vi "InitPIC.vi"(4 "error in (no error)":errorcluster, 6 "DeviceKey In":string, 7 "CmdLib In":refnum<k24>) -> (0 "error out":errorcluster, 1 "Device Address Out":i32, 2 "DeviceKey Out":string, 3 "CmdLib Out":refnum<k24>)   [LabVIEW 2018]
uses:
  Device VIs/CmdLib.dll
  Device VIs/Verbal.vi
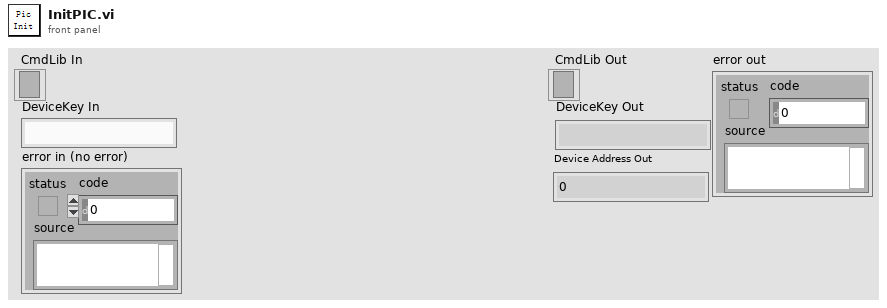
[diagram p1: front panel]
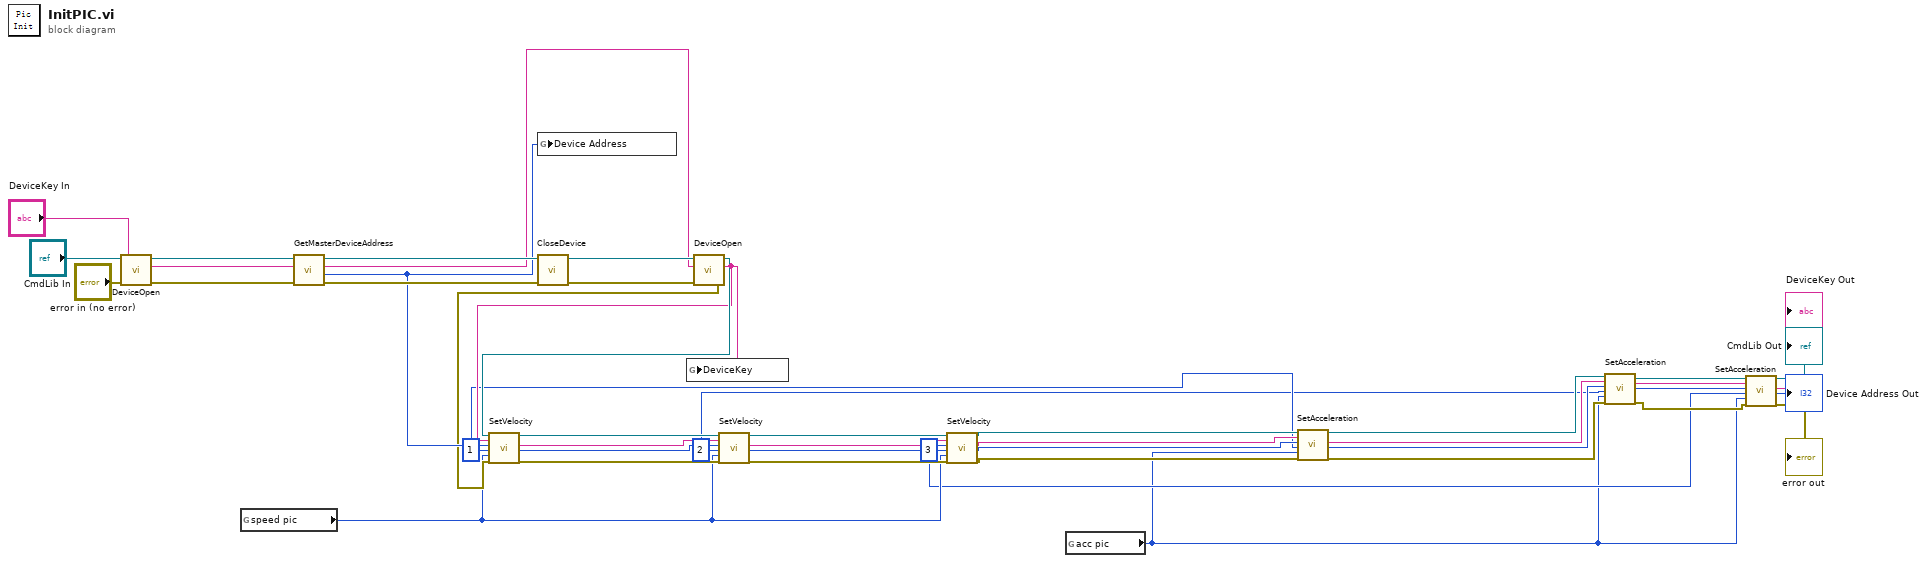
[diagram p0: block diagram]
diagram:
  w9 = 3 ("Motor")
  w14 = 2 ("Motor")
  w15 = 1 ("Motor")
  n1 = call "DeviceOpen.vi"("error in (no error)"="error in (no error)", "DeviceKey In"="DeviceKey In", "CmdLib In"="CmdLib In") -> ("error out"=w41:errorcluster, "DeviceKey Out"=w38:string, "CmdLib Out"=w42:refnum<k24>)  [unwired: 2 in]
  n2 = global read "Verbal.vi" "speed pic"() -> (w24:i32)
  n3 = call "GetMasterDeviceAddress.vi"("error in (no error)"=w41, "DeviceKey In"=w38, "CmdLib In"=w42) -> ("error out"=w39:errorcluster, "Device Address"=w26:i32, "DeviceKey Out"=w37:string, "CmdLib Out"=w40:refnum<k24>)  [unwired: 1 in]
  n4 = global write "Verbal.vi" "Device Address"(w26) -> ()
  n5 = call "CloseDevice.vi"("error in"=w39, "CmdLib In"=w40) -> ("error out"=w43:errorcluster, "CmdLib Out"=w44:refnum<k24>)  [unwired: 8 in]
  n6 = call "DeviceOpen.vi"("error in (no error)"=w43, "DeviceKey In"=w37, "CmdLib In"=w44) -> ("error out"=w25:errorcluster, "DeviceKey Out"=w27:string, "CmdLib Out"=w28:refnum<k24>)  [unwired: 2 in]
  n7 = call "SetVelocity.vi"("CmdLib In"=w28, "DeviceKey In"=w27, "Device Address In"=w26, "Motor"=w15, "Steps Per Sec"=w24, "error in (no error)"=w25) -> ("CmdLib Out"=w36:refnum<k24>, "DeviceKey Out"=w35:string, "Device Address Out"=w34:i32, "error out"=w33:errorcluster)  [unwired: 10 in]
  n8 = global write "Verbal.vi" "DeviceKey"(w27) -> ()
  n9 = call "SetVelocity.vi"("CmdLib In"=w36, "DeviceKey In"=w35, "Device Address In"=w34, "Motor"=w14, "Steps Per Sec"=w24, "error in (no error)"=w33) -> ("CmdLib Out"=w32:refnum<k24>, "DeviceKey Out"=w31:string, "Device Address Out"=w30:i32, "error out"=w29:errorcluster)  [unwired: 10 in]
  n10 = call "SetVelocity.vi"("CmdLib In"=w32, "DeviceKey In"=w31, "Device Address In"=w30, "Motor"=w9, "Steps Per Sec"=w24, "error in (no error)"=w29) -> ("CmdLib Out"=w19:refnum<k24>, "DeviceKey Out"=w18:string, "Device Address Out"=w17:i32, "error out"=w16:errorcluster)  [unwired: 10 in]
  n11 = global read "Verbal.vi" "acc pic"() -> (w8:i32)
  n12 = call "SetAcceleration.vi"("CmdLib In"=w19, "DeviceKey In"=w18, "Device Address In"=w17, "Motor"=w15, "Steps Per Sec 2"=w8, "error in (no error)"=w16) -> ("CmdLib Out"=w23:refnum<k24>, "DeviceKey Out"=w22:string, "Device Address Out"=w21:i32, "error out"=w20:errorcluster)  [unwired: 10 in]
  n13 = call "SetAcceleration.vi"("CmdLib In"=w23, "DeviceKey In"=w22, "Device Address In"=w21, "Motor"=w14, "Steps Per Sec 2"=w8, "error in (no error)"=w20) -> ("CmdLib Out"=w13:refnum<k24>, "DeviceKey Out"=w12:string, "Device Address Out"=w11:i32, "error out"=w10:errorcluster)  [unwired: 10 in]
  n14 = call "SetAcceleration.vi"("CmdLib In"=w13, "DeviceKey In"=w12, "Device Address In"=w11, "Motor"=w9, "Steps Per Sec 2"=w8, "error in (no error)"=w10) -> ("CmdLib Out"=→"CmdLib Out":refnum<k24>, "DeviceKey Out"=→"DeviceKey Out":string, "Device Address Out"=→"Device Address Out":i32, "error out"=→"error out":errorcluster)  [unwired: 10 in]
